vi "PortInt32_Get.vi"(8 "error in (no error)":errorcluster caption="错误输入（无错误）", 11 "Serial输入":refnum<class "Serial.lvclass">) -> (0 "error out":errorcluster caption="错误输出", 2 "端口-Int32":i32, 3 "Serial输出":refnum<class "Serial.lvclass">)   [LabVIEW 2012, in "Serial.lvclass"]
uses:
  Serial.lvclass
  Serial.lvclass/Serial.ctl
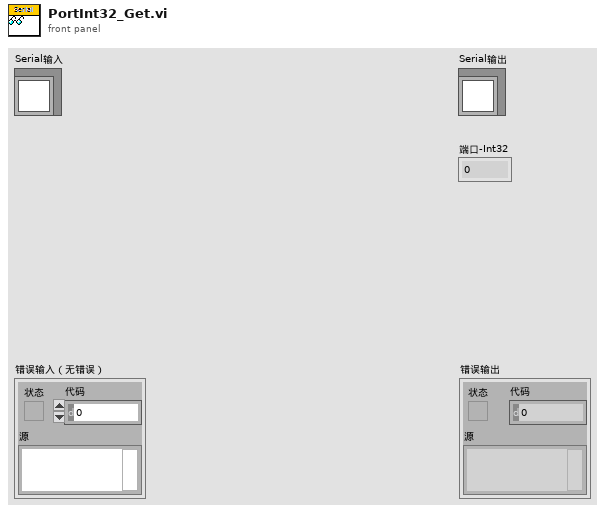
[diagram p1: front panel]
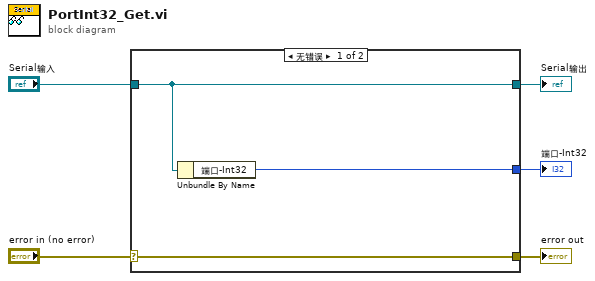
[diagram p0: block diagram]
diagram:
  n1 = case shown="无错误" "error in (no error)" {
    selector: "error in (no error)" -> [w8 w9]
    tunnel: [w8 w9] -> w4
    tunnel: [w7 w10] -> w2
    tunnel: "Serial输入" -> [w7 w10]
    tunnel: [w6 _] -> w1
    frame No Error {
      n2 = Unbundle By Name(w7) -> ("端口-Int32"=w6:i32)
    }
    frame Error {
    }
  }
  "error out" <- w4
  "Serial输出" <- w2
  "端口-Int32" <- w1
